vi "Check Out Reference.vi"(8 "error in (no error)":errorcluster, 11 "Shape Reference":refnum<data-value>) -> (0 "error out":errorcluster)   [LabVIEW 2017, in "LV Image Editor Framework.lvlib" / "Shape.lvclass"]
uses:
  Shape.lvclass
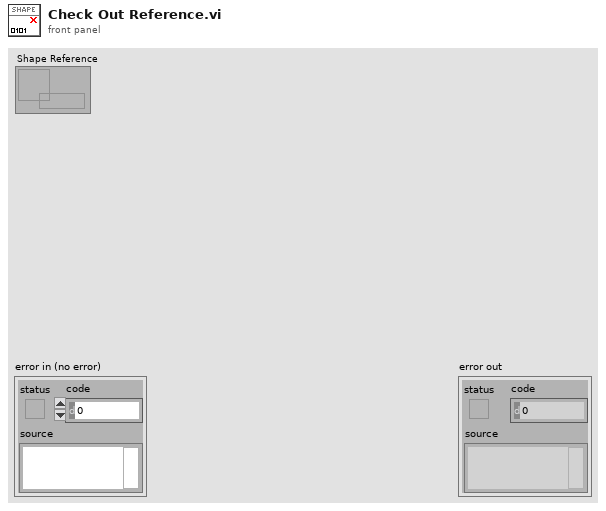
[diagram p1: front panel]
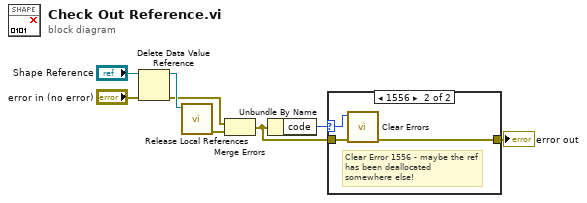
[diagram p0: block diagram]
diagram:
  n1 = Delete Data Value Reference(data value reference="Shape Reference", error in="error in (no error)") -> (data value=w6:refnum<class "Shape.lvclass">, error out=w5:errorcluster)
  n2 = call-dynamic "Release Local References.vi"("Shape in"=w6) -> ("error out"=w4:errorcluster)  [unwired: 10 in]
  n3 = Merge Errors(w5, w4) -> (w2:errorcluster)
  n4 = Unbundle By Name(w2) -> ("code"=w3:i32)
  n5 = case shown="1556" w3 {
    selector: w3 -> [_ w12]
    tunnel: w2 -> [w9 w11]
    tunnel: [w9 w10] -> w1
    frame Default {
    }
    frame 1556 {
      # "Clear Error 1556 - maybe the ref has been deallocated somewhere else!"
      n6 = call <vilib>:"Clear Errors.vi"("error in (no error)"=w11, "specific error code to clear (0: all)"=w12) -> ("error out"=w10:errorcluster)  [unwired: 4 in, 1 out]
    }
  }
  "error out" <- w1
